vi "PlaneFit.vi"(7 "Reset Clicks":bool, 8 "Y PEN":dbl, 9 "Z":dbl, 10 "Nano Z":dbl, 11 "X":dbl) -> (2 "Output":dbl, 3 "Clicks":dbl)   [LabVIEW 2019]
uses:
  <userlib>/HapticSTM/Feedbackless - Testdata/GlobalClicksHeight.vi
  <userlib>/HapticSTM/HapticSTM.lvlib
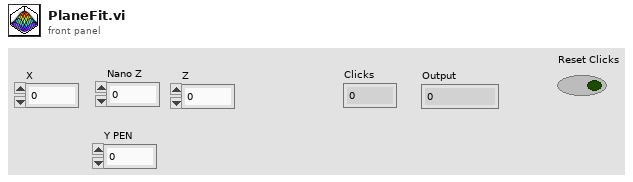
[diagram p1: front panel]
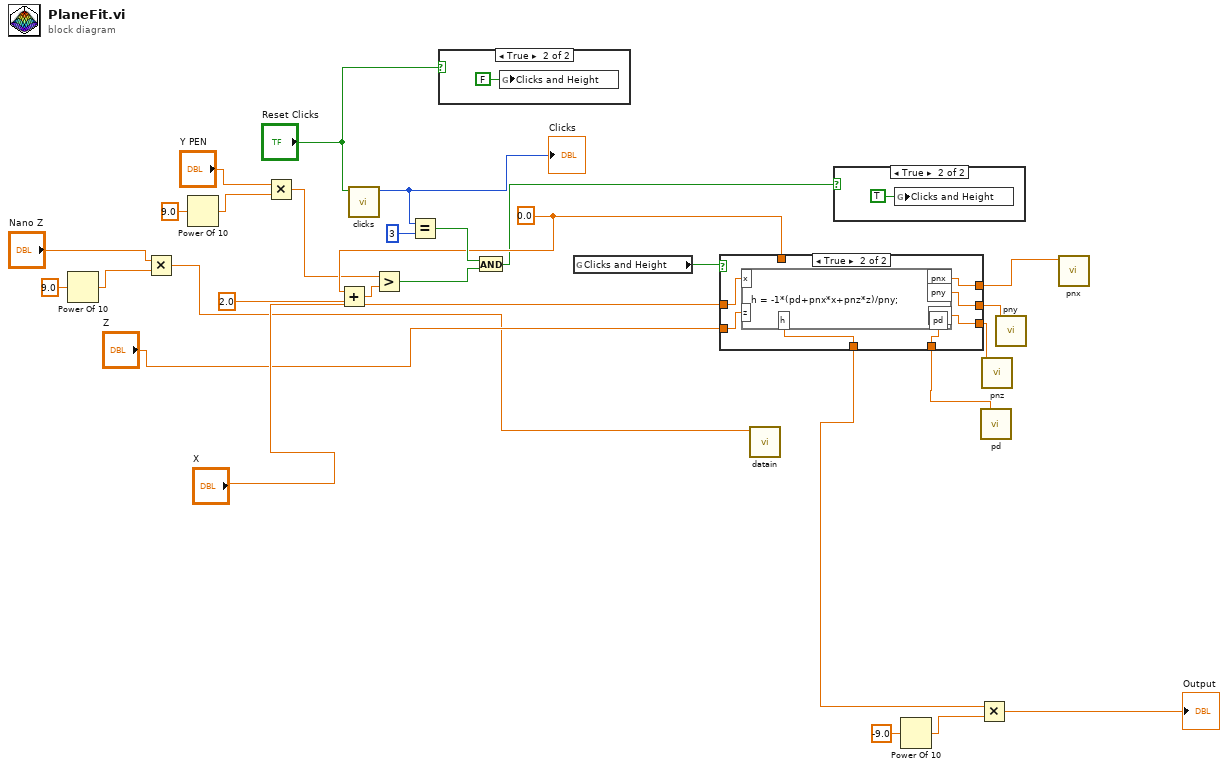
[diagram p0: block diagram]
diagram:
  w14 = 0.0 ("Plane Height")
  n1 = Power Of 10(x=9.0) -> (10^x=w6:dbl)
  n2 = Multiply(x="Nano Z", y=w6) -> (x*y=w1:dbl)
  n3 = Power Of 10(x=9.0) -> (10^x=w11:dbl)
  n4 = Multiply(x="Y PEN", y=w11) -> (x*y=w8:dbl)
  n5 = Add(x=w14, y=2.0) -> (x+y=w16:dbl)
  n6 = call <userlib>:"clicks.vi"("reset"="Reset Clicks") -> ("function return"=w26:i32)  [unwired: 10 in]
  "Clicks" <- w26
  n7 = Greater?(x=w8, y=w16) -> (0:w17:bool)
  n8 = Equal?(x=w26, y=3) -> (x = y?=w18:bool)
  n9 = case shown="True" "Reset Clicks" {
    frame False {
    }
    frame True {
      n10 = global write "GlobalClicksHeight.vi" "Clicks and Height"(FALSE ("Clicks and Height")) -> ()
    }
  }
  n11 = And(x=w18, y=w17) -> (x .and. y?=w13:bool)
  n12 = global read "GlobalClicksHeight.vi" "Clicks and Height"() -> (w12:bool)
  n13 = call <userlib>:"datain.vi"("output"=w1) -> ()  [unwired: 11 in]
  n14 = case shown="True" w13 {
    frame False {
    }
    frame True {
      n15 = global write "GlobalClicksHeight.vi" "Clicks and Height"(TRUE ("Clicks and Height")) -> ()
    }
  }
  n16 = Power Of 10(x=-9.0) -> (10^x=w21:dbl)
  n17 = call <userlib>:"pd.vi"() -> ("function return"=w27:dbl)  [unwired: 11 in]
  n18 = call <userlib>:"pnz.vi"() -> ("function return"=w28:dbl)  [unwired: 11 in]
  n19 = call <userlib>:"pny.vi"() -> ("function return"=w23:dbl)  [unwired: 11 in]
  n20 = call <userlib>:"pnx.vi"() -> ("function return"=w24:dbl)  [unwired: 11 in]
  n21 = case shown="True" w12 {
    tunnel: "X" -> [_ w38]
    tunnel: w24 -> [_ w36]
    tunnel: w23 -> [_ w35]
    tunnel: w28 -> [_ w34]
    tunnel: w27 -> [_ w33]
    tunnel: "Z" -> [_ w37]
    tunnel: [w31 w32] -> w2
    tunnel: w14 -> [w31 _]
    frame False {
    }
    frame True {
      n22 = formula code="h = -1*(pd+pnx*x+pnz*z)/pny;"("x"=w38, "z"=w37, "pnx"=w36, "pnz"=w34, "pd"=w33, "pny"=w35) -> ("h"=w32:dbl)
    }
  }
  n23 = Multiply(x=w2, y=w21) -> (x*y=→"Output":dbl)
